vi "miniproject.vi"() -> ()   [LabVIEW 2021]
uses:
  <vilib>/LabVIEW Interface for Arduino/LabVIEW Interface for Arduino.lvlib
panel:
  in  "SWITCH":bool
  out "STOP":bool
  out "RUN":bool
  in  "STOP":bool
  out "Tank":dbl(slide) scale=0.0..1000.0
  in  "Analog data in pin":u8
  in  "VISA resource":refnum<visa-resource-name>
  # "WATER LEVEL INDICATOR IN NI LABVEW  \nBY INTERFACING WITH ARDUINO"
  # "Volume = pi × radius² × height"
  # "FOR MANUAL OPERATION"
  # "1 Volt = 10mm = height"
  # "1 cm3 = 1 ml"
  # "1cm=10mm"
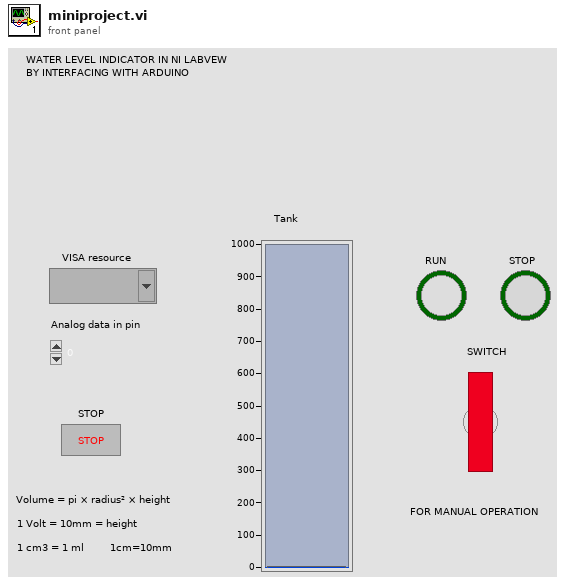
[diagram p1: front panel]
types:
  T1 = typedef "LabVIEW Interface for Arduino.lvlib/Arduino Resource.ctl" = cluster{"VISA resource":refnum<visa-resource-name>, "Board Type":T2, "Connection Type":enum8{"USB / Serial"}, "Bytes Per Packet (15)":u8}
  T2 = typedef "LabVIEW Interface for Arduino.lvlib/Board Type.ctl" = enum16{"Uno", "Dimuelanove w/Atmega 328", "Mega 2560"}
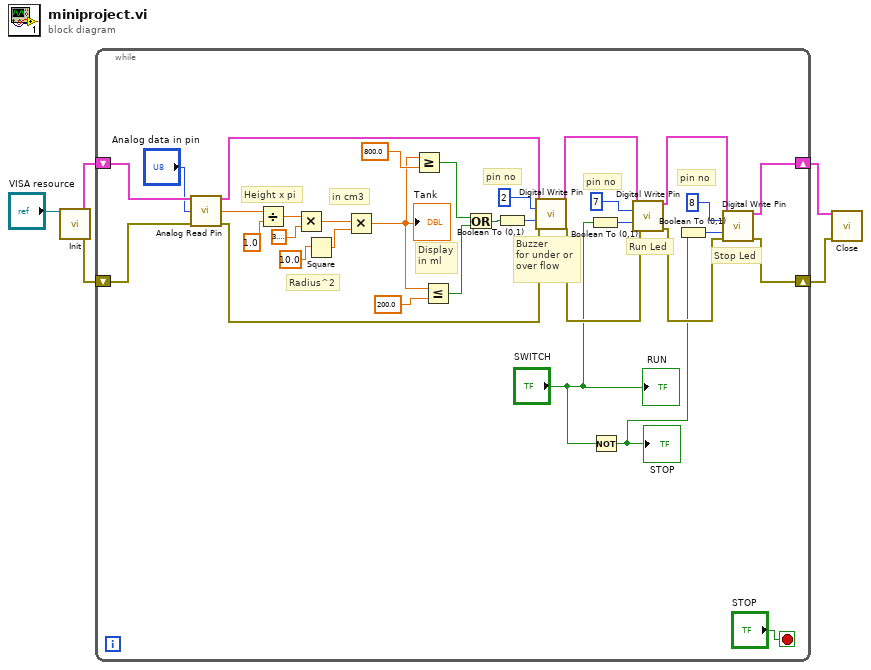
[diagram p0: block diagram]
diagram:
  n1 = call <vilib>:"Init.vi"("VISA resource"="VISA resource") -> ("Arduino Resource"=w4:T1, "error out"=w3:errorcluster)  [unwired: 17 in]
  n2 = while {
    shift-right: [w9] -> w2
    shift-left: w4 -> [w38]
    shift-right: [w8] -> w1
    shift-left: w3 -> [w37]
    stop <- "STOP" stop-if-true
    # "Stop Led"
    # "Run Led"
    # "Buzzer\nfor under or\nover flow"
    # "pin no"
    # "pin no"
    # "pin no"
    # "Display\nin ml"
    # "in cm3"
    # "Radius^2"
    # "Height x pi"
    n3 = call <vilib>:"Analog Read Pin.vi"("Arduino Resource"=w38, "Analog Input Pin (0)"="Analog data in pin", "error in"=w37) -> ("Arduino Resource"=w15:T1, "Voltage"=w34:dbl, "error out"=w14:errorcluster)  [unwired: 10 in]
    n4 = Divide(x=w34, y=1.0) -> (x/y=w32:dbl)
    n5 = Multiply(x=w32, y=3.141592653589793) -> (x*y=w30:dbl)
    n6 = Square(x=10.0) -> (x^2=w29:dbl)
    n7 = Multiply(x=w30, y=w29) -> (x*y=w16:dbl)
    "Tank" <- w16
    n8 = Greater Or Equal?(x=w16, y=800.0 ("x")) -> (x >= y?=w25:bool)
    n9 = Less Or Equal?(x=w16, y=200.0) -> (x <= y?=w24:bool)
    n10 = Or(x=w25, y=w24) -> (x .or. y?=w22:bool)
    n11 = Boolean To (0,1)(Boolean=w22) -> (0, 1=w21:i16)
    n12 = call <vilib>:"Digital Write Pin.vi"("Arduino Resource"=w15, "Digital I/O Pin (0)"=u8 2, "Value (0)"=w21, "error in"=w14) -> ("Arduino Resource"=w13:T1, "error out"=w12:errorcluster)  [unwired: 10 in]
    n13 = Boolean To (0,1)(Boolean="SWITCH") -> (0, 1=w17:i16)
    n14 = Not(x="SWITCH") -> (.not. x?=w6:bool)
    "STOP" <- w6
    n15 = call <vilib>:"Digital Write Pin.vi"("Arduino Resource"=w13, "Digital I/O Pin (0)"=u8 7, "Value (0)"=w17, "error in"=w12) -> ("Arduino Resource"=w11:T1, "error out"=w10:errorcluster)  [unwired: 10 in]
    n16 = Boolean To (0,1)(Boolean=w6) -> (0, 1=w18:i16)
    n17 = call <vilib>:"Digital Write Pin.vi"("Arduino Resource"=w11, "Digital I/O Pin (0)"=u8 8, "Value (0)"=w18, "error in"=w10) -> ("Arduino Resource"=w9:T1, "error out"=w8:errorcluster)  [unwired: 10 in]
    "RUN" <- "SWITCH"
  }
  n18 = call <vilib>:"Close.vi"("Arduino Resource"=w2, "error in"=w1) -> ()  [unwired: 13 in, 1 out]
